vi "Update Analog Output.vi"(6 "Simulate":bool, 8 "error in":errorcluster, 9 "timeout":dbl=10.0 format="%0.2f", 10 "AnalogVal in":dbl, 11 "AO Ref":refnum<k21>) -> (0 "error out":errorcluster, 1 "daqErr":bool, 3 "AO Ref out":refnum<k21>)   [LabVIEW 2017, in "DAQ.lvclass"]
doc: "Developed by Kevin Thompson\nThompson Engineering, LLC\nkevin@thompsonengineering.net"
uses:
  DAQ.lvclass
  <vilib>/DAQmx/write.llb/DAQmx Write (Analog DBL 1Chan 1Samp).vi
  <vilib>/DAQmx/miscellaneous.llb/DAQmx Fill In Error Info.vi
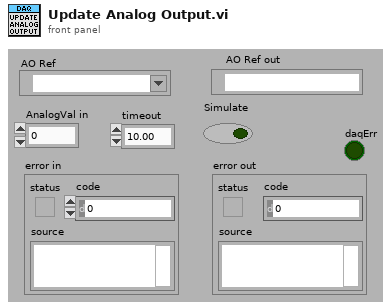
[diagram p1: front panel]
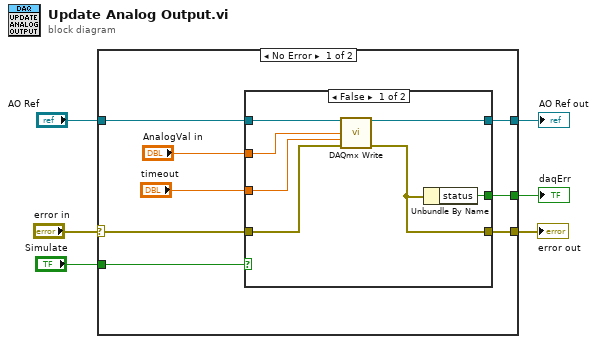
[diagram p0: block diagram]
diagram:
  n1 = case shown="No Error" "error in" {
    selector: "error in" -> [w9 w24]
    tunnel: "AO Ref" -> [w14 w25]
    tunnel: [w13 w25] -> w5
    tunnel: [w12 w24] -> w4
    tunnel: "Simulate" -> [w8 _]
    tunnel: [w7 _] -> w1
    frame No Error {
      n2 = case shown="False" w8 {
        tunnel: w14 -> [w21 w23]
        tunnel: [w20 w23] -> w13
        tunnel: [w16 w22] -> w12
        tunnel: "AnalogVal in" -> [w19 _]
        tunnel: "timeout" -> [w18 _]
        tunnel: w9 -> [w17 w22]
        tunnel: [w15 _] -> w7
        frame False {
          n3 = call-poly <vilib>:"DAQmx Write.vi"("task/channels in"=w21, "data"=w19, "timeout"=w18, "error in"=w17) -> ("task out"=w20:refnum<k21>, "error out"=w16:errorcluster)  [unwired: 9 in, 1 out]
          n4 = Unbundle By Name(w16) -> ("status"=w15:bool)
        }
        frame True {
        }
      }
    }
    frame Error {
    }
  }
  "error out" <- w4
  "AO Ref out" <- w5
  "daqErr" <- w1
